vi "Auto Watchdog.vi"(1 "Motor Input":dbl, 2 "Velocity":dbl format="%#_13g") -> (0 "Output":bool)   [LabVIEW 2015]
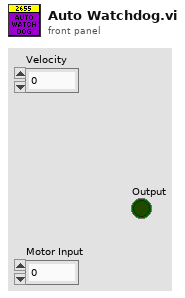
[diagram p1: front panel]
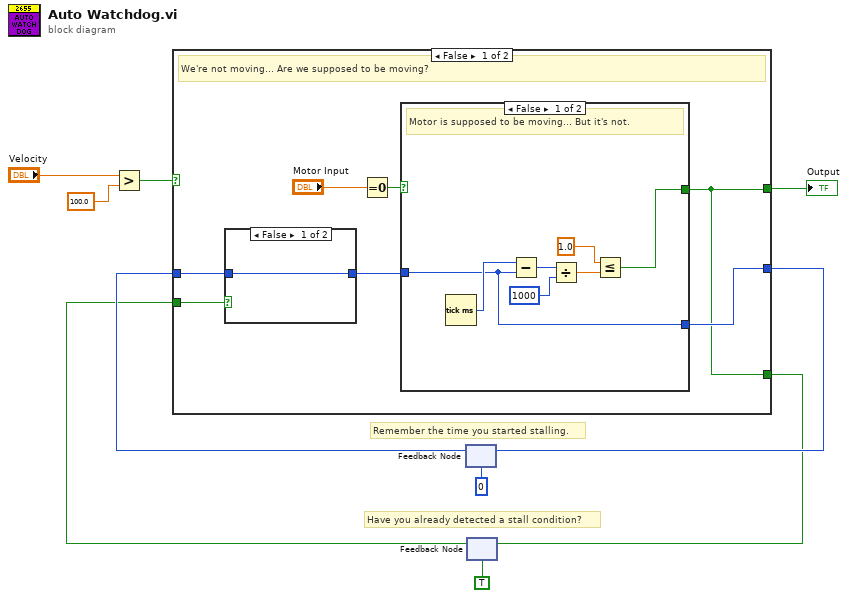
[diagram p0: block diagram]
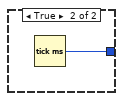
[diagram p2: hidden frame]
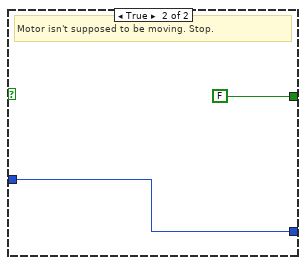
[diagram p3: hidden frame]
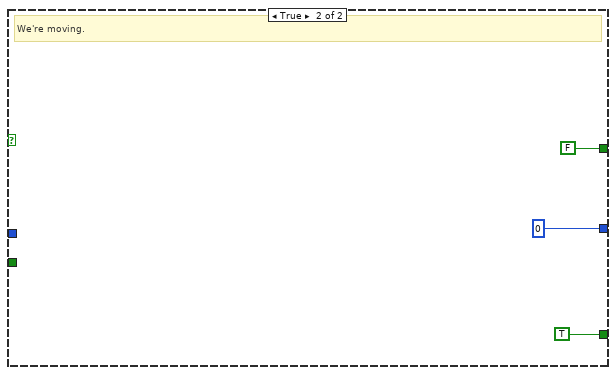
[diagram p4: hidden frame]
diagram:
  # "Have you already detected a stall condition?"
  # "Remember the time you started stalling."
  n1 = Greater?(x="Velocity", y=100.0) -> (0:w8:bool)
  n2 = feedback #1(u32 0 ("millisecond timer value")) -> (w6:u32)
  n3 = feedback #2(TRUE ("f")) -> (w1:bool)
  n4 = case shown="False" w8 {
    tunnel: [w11 FALSE ("f")] -> w7
    tunnel: w6 -> [w14 _]
    tunnel: [w15 0] -> w5
    tunnel: [w11 TRUE ("f")] -> w2
    tunnel: w1 -> [w12 _]
    frame False {
      # "We're not moving... Are we supposed to be moving?"
      n5 = case shown="False" w12 {
        tunnel: [w18 w19] -> w13
        tunnel: w14 -> [w18 _]
        frame False {
        }
        frame True {
          n6 = Tick Count (ms)() -> (millisecond timer value=w19:u32)
        }
      }
      n7 = Equal To 0?(x="Motor Input") -> (x = 0?=w16:bool)
      n8 = case shown="False" w16 {
        tunnel: [w21 FALSE ("f")] -> w11
        tunnel: w13 -> [w20 w27]
        tunnel: [w20 w27] -> w15
        frame False {
          # "Motor is supposed to be moving... But it's not."
          n9 = Tick Count (ms)() -> (millisecond timer value=w26:u32)
          n10 = Subtract(x=w26, y=w20) -> (x-y=w25:u32)
          n11 = Divide(x=w25, y=u32 1000) -> (x/y=w23:dbl)
          n12 = Less Or Equal?(x=1.0, y=w23) -> (x <= y?=w21:bool)
        }
        frame True {
          # "Motor isn't supposed to be moving. Stop."
        }
      }
    }
    frame True {
      # "We're moving."
    }
  }
  "Output" <- w7
  n13 = feedback-in #1(w5) -> ()
  n14 = feedback-in #2(w2) -> ()
